vi "sum.vi"(9 "y":dbl, 10 "x":dbl, 11 "Calculator in":refnum<class "Calculator.lvclass">) -> (2 "x+y":dbl, 3 "Calculator out":refnum<class "Calculator.lvclass">)   [LabVIEW 2018, in "Calculator.lvclass"]
doc: "[Covers: ADD_REQ1]"
uses:
  Calculator.lvclass
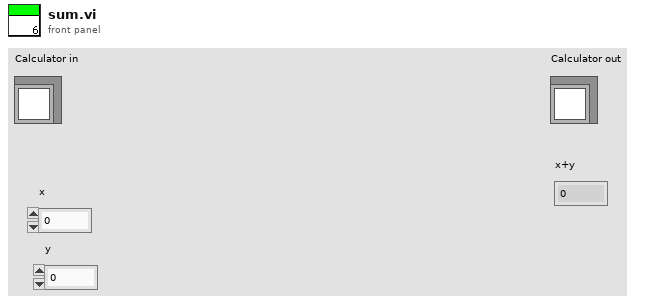
[diagram p1: front panel]
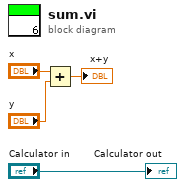
[diagram p0: block diagram]
diagram:
  n1 = Add(x="x", y="y") -> (x+y=→"x+y":dbl)
  "Calculator out" <- "Calculator in"
